vi "sub_Format Rx Data.vi"(1 "Array":dbl[](array[numeric])) -> (0 "Received Message":string)   [LabVIEW 2014]
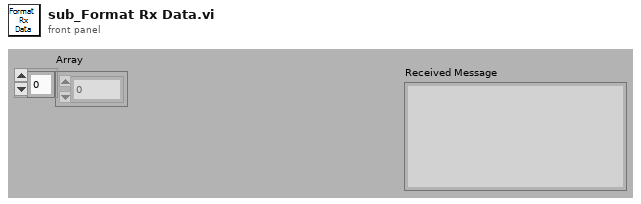
[diagram p1: front panel]
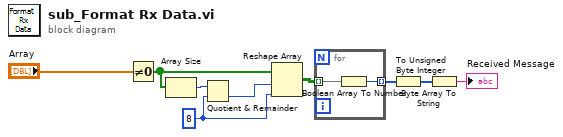
[diagram p0: block diagram]
diagram:
  w5 = 8 ("dimension size")
  n1 = Not Equal To 0?(x="Array") -> (x != 0?=w3:bool[])
  n2 = Array Size(array=w3) -> (size(s)=w4:i32)
  n3 = Quotient & Remainder(x=w4, y=w5) -> (floor(x/y)=w2:i32)  [unwired: 1 out]
  n4 = Reshape Array(w3, w2, w5) -> (w6:bool[][])
  n5 = for {
    tunnel: w6 -> [w11] mode=indexing
    tunnel: [w10] -> w7 mode=indexing
    n6 = Boolean Array To Number(Boolean array=w11) -> (number=w10:u32)
  }
  n7 = To Unsigned Byte Integer(number=w7) -> (unsigned 8bit integer=w8:u8[])
  n8 = Byte Array To String(unsigned byte array=w8) -> (string=→"Received Message":string)
